vi "Configure.vi"(8 "error in (no error)":errorcluster, 9 "Default Path":path, 10 "Interactive?":bool, 11 "Report Interface in":refnum<class "Report Interface.lvclass">) -> (0 "error out":errorcluster, 3 "Report Interface out":refnum<class "Report Interface.lvclass">)   [LabVIEW 2020, in "Report Interface.lvclass"]
uses:
  Report Interface.lvclass
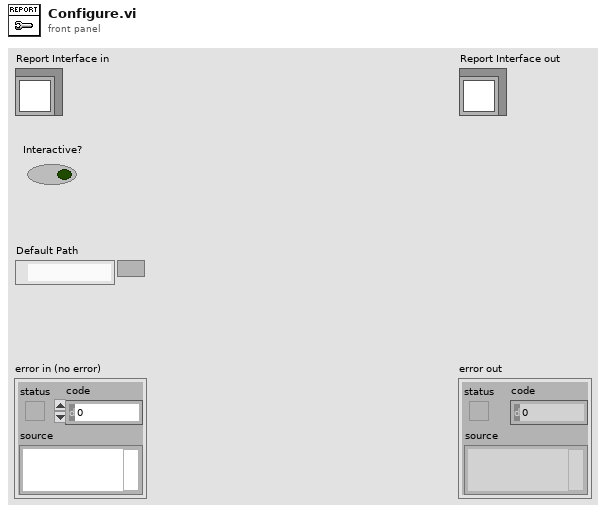
[diagram p1: front panel]
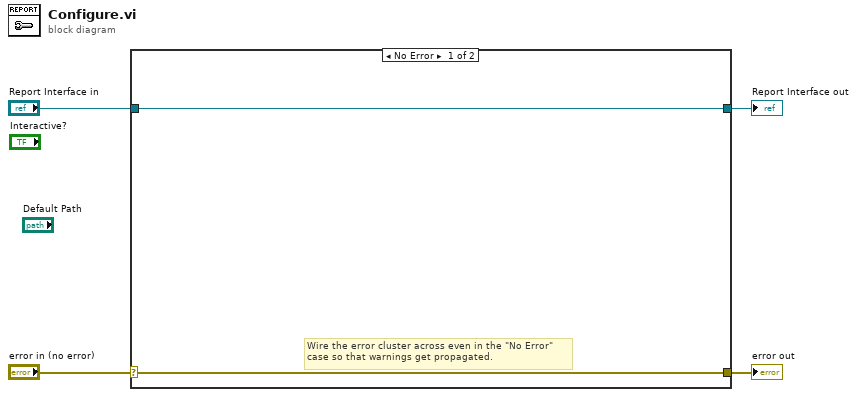
[diagram p0: block diagram]
diagram:
  n1 = case shown="No Error" "error in (no error)" {
    selector: "error in (no error)" -> [w5 w8]
    tunnel: [w5 w8] -> w3
    tunnel: [w6 w7] -> w1
    tunnel: "Report Interface in" -> [w6 w7]
    frame No Error {
      # "Wire the error cluster across even in the \"No Error\"\ncase so that warnings get propagated."
    }
    frame Error {
    }
  }
  "error out" <- w3
  "Report Interface out" <- w1
